vi "GetAllAnalogInputVals.vi"(8 "error in (no error)":errorcluster, 11 "SerialPortRef":T1) -> (0 "error out":errorcluster, 1 "ADC raw values":u32[](array[numeric]) format="%012b", 2 "ADC voltages":dbl[](array[numeric]), 3 "SerialPortRef 2":T1)   [LabVIEW 2015]
uses:
  <vilib>/Rock Robotics/WPI/SerialPort/WPI_SerialPortRef.ctl
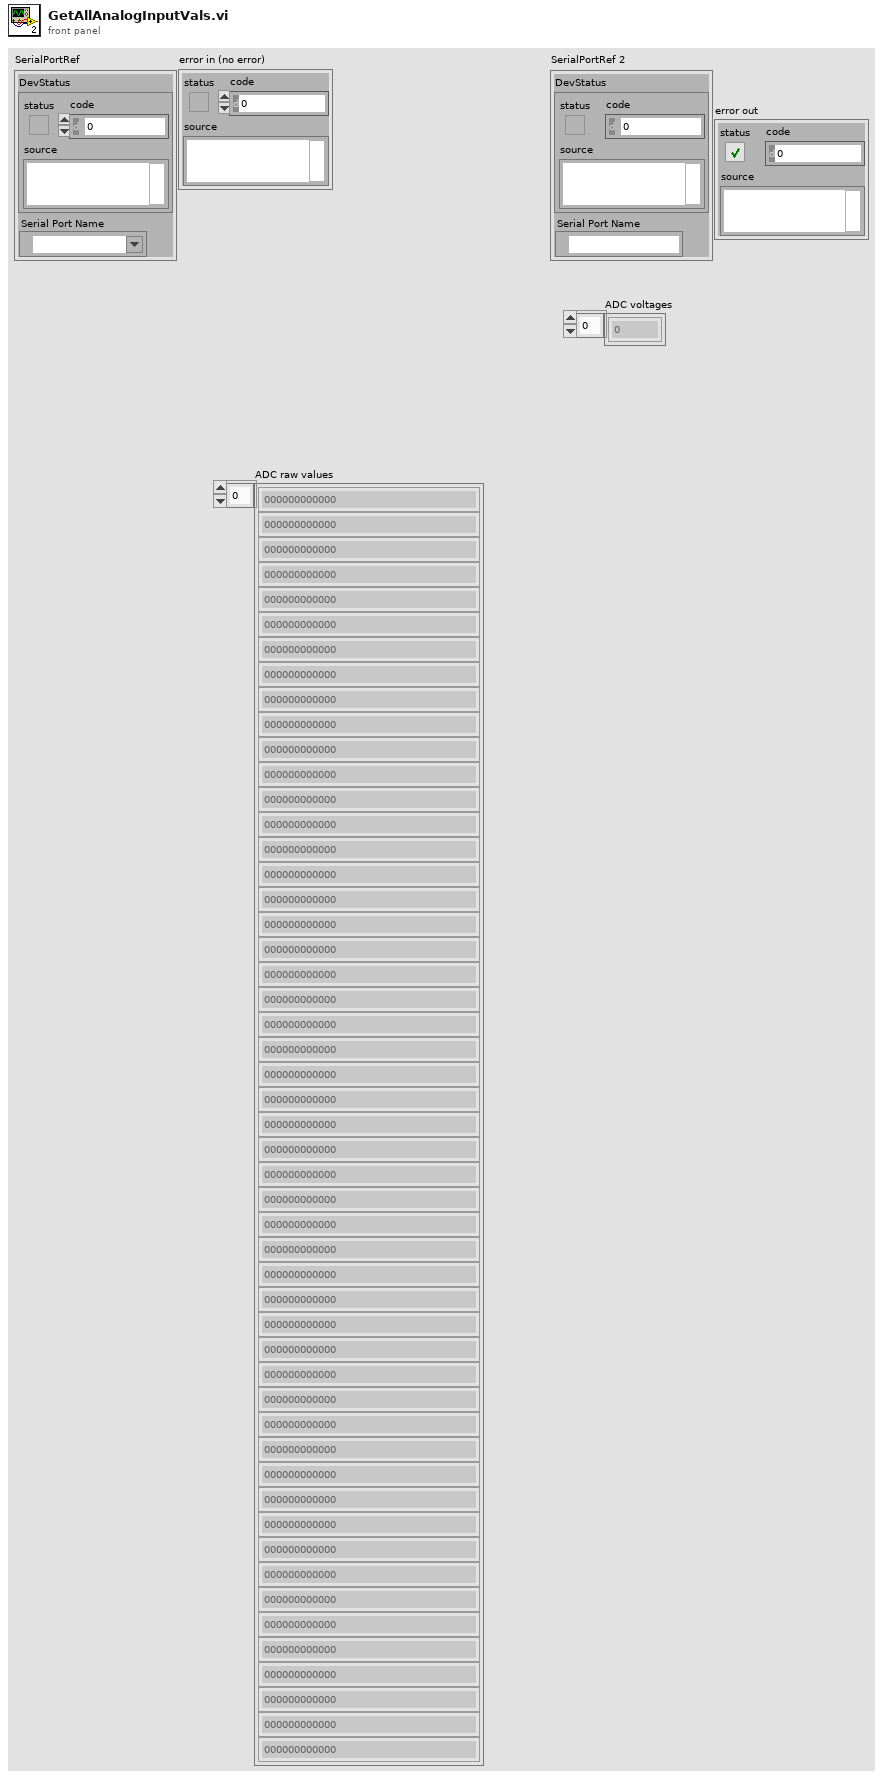
[diagram p1: front panel]
types:
  T1 = typedef "WPI_SerialPortRef.ctl" = cluster{"DevStatus":errorcluster, "Serial Port Name":refnum<visa-resource-name>}
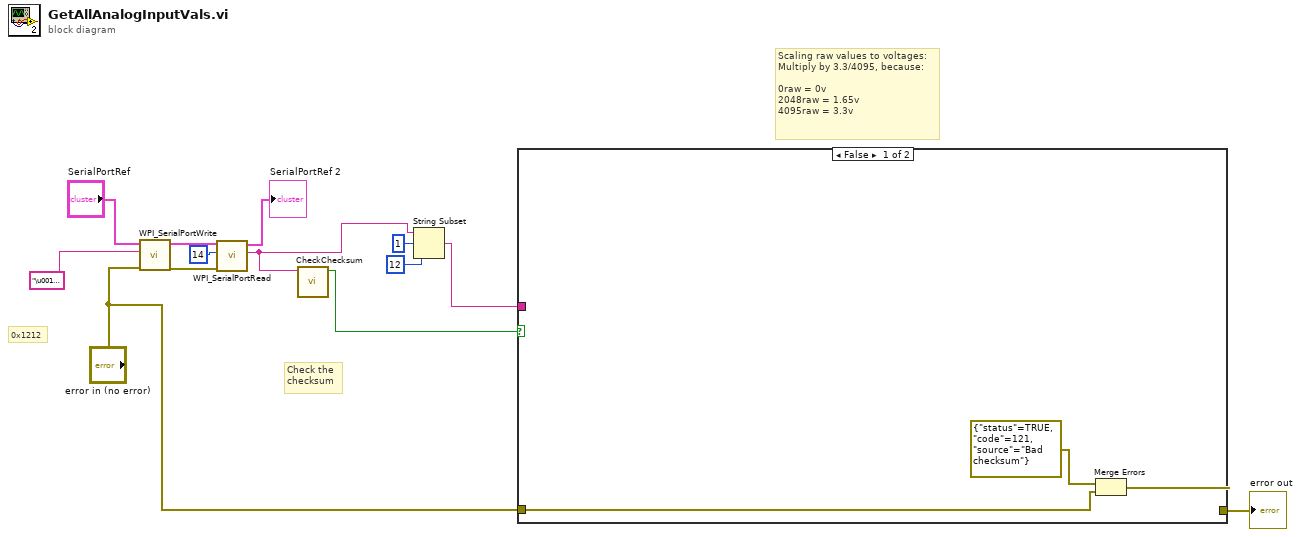
[diagram p0: block diagram]
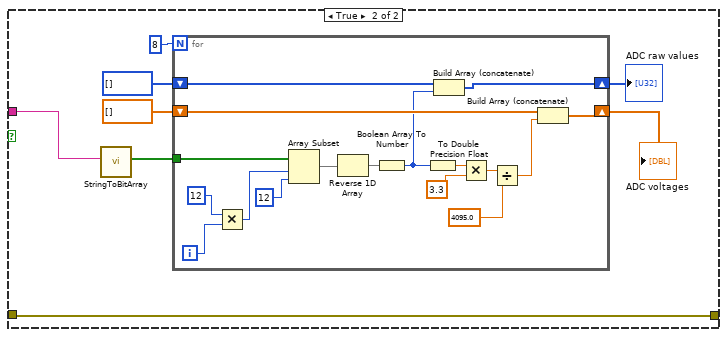
[diagram p2: hidden frame]
diagram:
  # "Scaling raw values to voltages:\nMultiply by 3.3/4095, because:\n\n0raw = 0v\n2048raw = 1.65v\n4095raw = 3.3v"
  # "Check the\nchecksum"
  # "0x1212"
  n1 = call <vilib>:"WPI_SerialPortWrite.vi"("error in (no error)"="error in (no error)", "Buffer"="\u0012\u0012", "SerialPortRef"="SerialPortRef") -> ("error out"=w4:errorcluster, "SerialPortRef"=w5:T1)  [unwired: 6 in, 1 out]
  n2 = call <vilib>:"WPI_SerialPortRead.vi"("error in (no error)"=w4, "Num Bytes to Read"=u32 14, "SerialPortRef"=w5) -> ("Buffer"=w2:string, "SerialPortRef"=→"SerialPortRef 2":T1)  [unwired: 6 in, 1 out]
  n3 = call "CheckChecksum.vi"("String"=w2) -> ("x = y?"=w1:bool)  [unwired: 10 in]
  n4 = String Subset(string=w2, offset (0)=1, length (rest)=12 ("length (rest)")) -> (substring=w9:string)
  n5 = case shown="False" w1 {
    tunnel: w9 -> [_ w19]
    tunnel: "error in (no error)" -> [w15 w24]
    tunnel: [w14 w24] -> w8
    frame False {
      n6 = Merge Errors(errorcluster {"status"=TRUE, "code"=121, "source"="Bad checksum"} ("error in"), w15) -> (w14:errorcluster)
    }
    frame True {
      n7 = call "StringToBitArray.vi"("string"=w19) -> ("Array"=w22:bool[])  [unwired: 10 in]
      n8 = for {
        N: 8 -> [_]
        tunnel: w22 -> [w41]
        shift-right: [w37] -> w20
        shift-left: u32[] [] -> [w36]
        shift-right: [w32] -> w17
        shift-left: dbl[] [] -> [w31]
        i -> [w40]
        n9 = Multiply(x=12, y=w40) -> (x*y=w38:i32)
        n10 = Array Subset(array=w41, index=w38, length=12) -> (w34:bool[])
        n11 = Reverse 1D Array(array=w34) -> (reversed array=w33:bool[])
        n12 = Boolean Array To Number(Boolean array=w33) -> (number=w25:u32)
        n13 = To Double Precision Float(number=w25) -> (double precision float=w26:dbl)
        n14 = Build Array (concatenate)(w36, w25) -> (w37:u32[])
        n15 = Multiply(x=w26, y=3.3) -> (x*y=w29:dbl)
        n16 = Divide(x=w29, y=4095.0) -> (x/y=w27:dbl)
        n17 = Build Array (concatenate)(w31, w27) -> (w32:dbl[])
      }
      "ADC raw values" <- w20
      "ADC voltages" <- w17
    }
  }
  "error out" <- w8
